vi "Simple Wait.vi"(0 "Bool In":bool, 7 "mS":u32, 11 "error in":errorcluster) -> (4 "Bool Out":bool, 15 "error out":errorcluster)   [LabVIEW 2020]
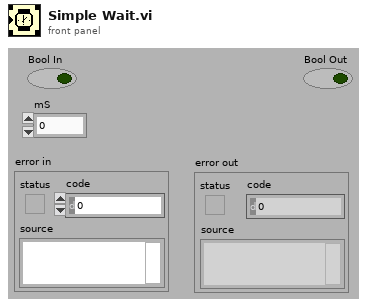
[diagram p1: front panel]
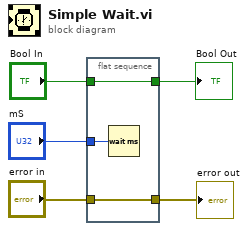
[diagram p0: block diagram]
diagram:
  n1 = flat-sequence {
    tunnel: "error in" -> [w8]
    tunnel: [w8] -> w4
    tunnel: "Bool In" -> [w7]
    tunnel: [w7] -> w1
    tunnel: "mS" -> [w6]
    frame #0 {
      n2 = Wait (ms)(milliseconds to wait=w6) -> ()  [unwired: 1 out]
    }
  }
  "error out" <- w4
  "Bool Out" <- w1
